vi "2b_state_sel.vi"(9 "keys pressed":T1(array[ring]), 10 "down/back":dbl, 11 "up/fwd":dbl) -> (2 "down/back":bool, 3 "up/fwd":bool)   [LabVIEW 2012]
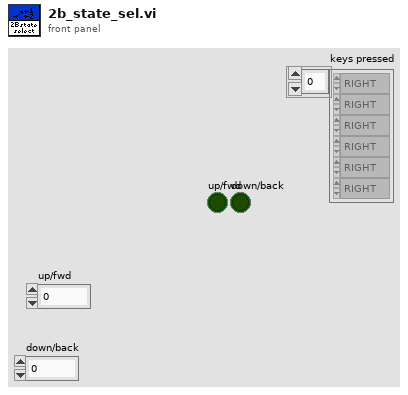
[diagram p1: front panel]
types:
  T1 = enum16{"0", "1", "2", "3", "4", "5", "6", "7", "8", "9", "A", "B", "C", "D", "E", "F", "G", "H", "I", "J", "K", "L", "M", "N", "O", "P", "Q", "R", "S", "T", "U", "V", "W", "X", "Y", "Z", "F1", "F2", "F3", "F4", "F5", "F6", "F7", "F8", "F9", "F10", "F11", "F12", "F13", "F14", "F15", "ADD", "BACK", "BACKSLASH", "CAPITAL", "COMMA", "DECIMAL", "DELETE", "DIVIDE", "DOWN", "END", "EQUALS", "ESCAPE", "GRAVE (`)", "HOME", "INSERT", "LBRACKET", "LCONTROL", "LEFT", "L ALT", "LSHIFT", "LWIN", "MINUS", "MULTIPLY", "NEXT", "NUMLOCK", "NUMPAD_0", "NUMPAD_1", "NUMPAD_2", "NUMPAD_3", "NUMPAD_4", "NUMPAD_5", "NUMPAD_6", "NUMPAD_7", "NUMPAD_8", "NUMPAD_9", "PAUSE", "PERIOD", "PRIOR (PG UP)", "RBRACKET", "RCONTROL", "RETURN", "RIGHT", "R ALT", "RSHIFT", "RWIN", "SCROLL", "SEMICOLON", "SLASH", "SPACE", "SUBTRACT", "TAB", "UP", "ENTER (num pad)", "' (quote)"}[]
  T2 = cluster{"keys pressed[0]":enum16{"0", "1", "2", "3", "4", "5", "6", "7", "8", "9", "A", "B", "C", "D", "E", "F", "G", "H", "I", "J", "K", "L", "M", "N", "O", "P", "Q", "R", "S", "T", "U", "V", "W", "X", "Y", "Z", "F1", "F2", "F3", "F4", "F5", "F6", "F7", "F8", "F9", "F10", "F11", "F12", "F13", "F14", "F15", "ADD", "BACK", "BACKSLASH", "CAPITAL", "COMMA", "DECIMAL", "DELETE", "DIVIDE", "DOWN", "END", "EQUALS", "ESCAPE", "GRAVE (`)", "HOME", "INSERT", "LBRACKET", "LCONTROL", "LEFT", "L ALT", "LSHIFT", "LWIN", "MINUS", "MULTIPLY", "NEXT", "NUMLOCK", "NUMPAD_0", "NUMPAD_1", "NUMPAD_2", "NUMPAD_3", "NUMPAD_4", "NUMPAD_5", "NUMPAD_6", "NUMPAD_7", "NUMPAD_8", "NUMPAD_9", "PAUSE", "PERIOD", "PRIOR (PG UP)", "RBRACKET", "RCONTROL", "RETURN", "RIGHT", "R ALT", "RSHIFT", "RWIN", "SCROLL", "SEMICOLON", "SLASH", "SPACE", "SUBTRACT", "TAB", "UP", "ENTER (num pad)", "' (quote)"}, "keys pressed[1]":enum16{"0", "1", "2", "3", "4", "5", "6", "7", "8", "9", "A", "B", "C", "D", "E", "F", "G", "H", "I", "J", "K", "L", "M", "N", "O", "P", "Q", "R", "S", "T", "U", "V", "W", "X", "Y", "Z", "F1", "F2", "F3", "F4", "F5", "F6", "F7", "F8", "F9", "F10", "F11", "F12", "F13", "F14", "F15", "ADD", "BACK", "BACKSLASH", "CAPITAL", "COMMA", "DECIMAL", "DELETE", "DIVIDE", "DOWN", "END", "EQUALS", "ESCAPE", "GRAVE (`)", "HOME", "INSERT", "LBRACKET", "LCONTROL", "LEFT", "L ALT", "LSHIFT", "LWIN", "MINUS", "MULTIPLY", "NEXT", "NUMLOCK", "NUMPAD_0", "NUMPAD_1", "NUMPAD_2", "NUMPAD_3", "NUMPAD_4", "NUMPAD_5", "NUMPAD_6", "NUMPAD_7", "NUMPAD_8", "NUMPAD_9", "PAUSE", "PERIOD", "PRIOR (PG UP)", "RBRACKET", "RCONTROL", "RETURN", "RIGHT", "R ALT", "RSHIFT", "RWIN", "SCROLL", "SEMICOLON", "SLASH", "SPACE", "SUBTRACT", "TAB", "UP", "ENTER (num pad)", "' (quote)"}, "keys pressed[2]":enum16{"0", "1", "2", "3", "4", "5", "6", "7", "8", "9", "A", "B", "C", "D", "E", "F", "G", "H", "I", "J", "K", "L", "M", "N", "O", "P", "Q", "R", "S", "T", "U", "V", "W", "X", "Y", "Z", "F1", "F2", "F3", "F4", "F5", "F6", "F7", "F8", "F9", "F10", "F11", "F12", "F13", "F14", "F15", "ADD", "BACK", "BACKSLASH", "CAPITAL", "COMMA", "DECIMAL", "DELETE", "DIVIDE", "DOWN", "END", "EQUALS", "ESCAPE", "GRAVE (`)", "HOME", "INSERT", "LBRACKET", "LCONTROL", "LEFT", "L ALT", "LSHIFT", "LWIN", "MINUS", "MULTIPLY", "NEXT", "NUMLOCK", "NUMPAD_0", "NUMPAD_1", "NUMPAD_2", "NUMPAD_3", "NUMPAD_4", "NUMPAD_5", "NUMPAD_6", "NUMPAD_7", "NUMPAD_8", "NUMPAD_9", "PAUSE", "PERIOD", "PRIOR (PG UP)", "RBRACKET", "RCONTROL", "RETURN", "RIGHT", "R ALT", "RSHIFT", "RWIN", "SCROLL", "SEMICOLON", "SLASH", "SPACE", "SUBTRACT", "TAB", "UP", "ENTER (num pad)", "' (quote)"}, "keys pressed[3]":enum16{"0", "1", "2", "3", "4", "5", "6", "7", "8", "9", "A", "B", "C", "D", "E", "F", "G", "H", "I", "J", "K", "L", "M", "N", "O", "P", "Q", "R", "S", "T", "U", "V", "W", "X", "Y", "Z", "F1", "F2", "F3", "F4", "F5", "F6", "F7", "F8", "F9", "F10", "F11", "F12", "F13", "F14", "F15", "ADD", "BACK", "BACKSLASH", "CAPITAL", "COMMA", "DECIMAL", "DELETE", "DIVIDE", "DOWN", "END", "EQUALS", "ESCAPE", "GRAVE (`)", "HOME", "INSERT", "LBRACKET", "LCONTROL", "LEFT", "L ALT", "LSHIFT", "LWIN", "MINUS", "MULTIPLY", "NEXT", "NUMLOCK", "NUMPAD_0", "NUMPAD_1", "NUMPAD_2", "NUMPAD_3", "NUMPAD_4", "NUMPAD_5", "NUMPAD_6", "NUMPAD_7", "NUMPAD_8", "NUMPAD_9", "PAUSE", "PERIOD", "PRIOR (PG UP)", "RBRACKET", "RCONTROL", "RETURN", "RIGHT", "R ALT", "RSHIFT", "RWIN", "SCROLL", "SEMICOLON", "SLASH", "SPACE", "SUBTRACT", "TAB", "UP", "ENTER (num pad)", "' (quote)"}, "keys pressed[4]":enum16{"0", "1", "2", "3", "4", "5", "6", "7", "8", "9", "A", "B", "C", "D", "E", "F", "G", "H", "I", "J", "K", "L", "M", "N", "O", "P", "Q", "R", "S", "T", "U", "V", "W", "X", "Y", "Z", "F1", "F2", "F3", "F4", "F5", "F6", "F7", "F8", "F9", "F10", "F11", "F12", "F13", "F14", "F15", "ADD", "BACK", "BACKSLASH", "CAPITAL", "COMMA", "DECIMAL", "DELETE", "DIVIDE", "DOWN", "END", "EQUALS", "ESCAPE", "GRAVE (`)", "HOME", "INSERT", "LBRACKET", "LCONTROL", "LEFT", "L ALT", "LSHIFT", "LWIN", "MINUS", "MULTIPLY", "NEXT", "NUMLOCK", "NUMPAD_0", "NUMPAD_1", "NUMPAD_2", "NUMPAD_3", "NUMPAD_4", "NUMPAD_5", "NUMPAD_6", "NUMPAD_7", "NUMPAD_8", "NUMPAD_9", "PAUSE", "PERIOD", "PRIOR (PG UP)", "RBRACKET", "RCONTROL", "RETURN", "RIGHT", "R ALT", "RSHIFT", "RWIN", "SCROLL", "SEMICOLON", "SLASH", "SPACE", "SUBTRACT", "TAB", "UP", "ENTER (num pad)", "' (quote)"}, "keys pressed[5]":enum16{"0", "1", "2", "3", "4", "5", "6", "7", "8", "9", "A", "B", "C", "D", "E", "F", "G", "H", "I", "J", "K", "L", "M", "N", "O", "P", "Q", "R", "S", "T", "U", "V", "W", "X", "Y", "Z", "F1", "F2", "F3", "F4", "F5", "F6", "F7", "F8", "F9", "F10", "F11", "F12", "F13", "F14", "F15", "ADD", "BACK", "BACKSLASH", "CAPITAL", "COMMA", "DECIMAL", "DELETE", "DIVIDE", "DOWN", "END", "EQUALS", "ESCAPE", "GRAVE (`)", "HOME", "INSERT", "LBRACKET", "LCONTROL", "LEFT", "L ALT", "LSHIFT", "LWIN", "MINUS", "MULTIPLY", "NEXT", "NUMLOCK", "NUMPAD_0", "NUMPAD_1", "NUMPAD_2", "NUMPAD_3", "NUMPAD_4", "NUMPAD_5", "NUMPAD_6", "NUMPAD_7", "NUMPAD_8", "NUMPAD_9", "PAUSE", "PERIOD", "PRIOR (PG UP)", "RBRACKET", "RCONTROL", "RETURN", "RIGHT", "R ALT", "RSHIFT", "RWIN", "SCROLL", "SEMICOLON", "SLASH", "SPACE", "SUBTRACT", "TAB", "UP", "ENTER (num pad)", "' (quote)"}, "keys pressed[6]":enum16{"0", "1", "2", "3", "4", "5", "6", "7", "8", "9", "A", "B", "C", "D", "E", "F", "G", "H", "I", "J", "K", "L", "M", "N", "O", "P", "Q", "R", "S", "T", "U", "V", "W", "X", "Y", "Z", "F1", "F2", "F3", "F4", "F5", "F6", "F7", "F8", "F9", "F10", "F11", "F12", "F13", "F14", "F15", "ADD", "BACK", "BACKSLASH", "CAPITAL", "COMMA", "DECIMAL", "DELETE", "DIVIDE", "DOWN", "END", "EQUALS", "ESCAPE", "GRAVE (`)", "HOME", "INSERT", "LBRACKET", "LCONTROL", "LEFT", "L ALT", "LSHIFT", "LWIN", "MINUS", "MULTIPLY", "NEXT", "NUMLOCK", "NUMPAD_0", "NUMPAD_1", "NUMPAD_2", "NUMPAD_3", "NUMPAD_4", "NUMPAD_5", "NUMPAD_6", "NUMPAD_7", "NUMPAD_8", "NUMPAD_9", "PAUSE", "PERIOD", "PRIOR (PG UP)", "RBRACKET", "RCONTROL", "RETURN", "RIGHT", "R ALT", "RSHIFT", "RWIN", "SCROLL", "SEMICOLON", "SLASH", "SPACE", "SUBTRACT", "TAB", "UP", "ENTER (num pad)", "' (quote)"}, "keys pressed[7]":enum16{"0", "1", "2", "3", "4", "5", "6", "7", "8", "9", "A", "B", "C", "D", "E", "F", "G", "H", "I", "J", "K", "L", "M", "N", "O", "P", "Q", "R", "S", "T", "U", "V", "W", "X", "Y", "Z", "F1", "F2", "F3", "F4", "F5", "F6", "F7", "F8", "F9", "F10", "F11", "F12", "F13", "F14", "F15", "ADD", "BACK", "BACKSLASH", "CAPITAL", "COMMA", "DECIMAL", "DELETE", "DIVIDE", "DOWN", "END", "EQUALS", "ESCAPE", "GRAVE (`)", "HOME", "INSERT", "LBRACKET", "LCONTROL", "LEFT", "L ALT", "LSHIFT", "LWIN", "MINUS", "MULTIPLY", "NEXT", "NUMLOCK", "NUMPAD_0", "NUMPAD_1", "NUMPAD_2", "NUMPAD_3", "NUMPAD_4", "NUMPAD_5", "NUMPAD_6", "NUMPAD_7", "NUMPAD_8", "NUMPAD_9", "PAUSE", "PERIOD", "PRIOR (PG UP)", "RBRACKET", "RCONTROL", "RETURN", "RIGHT", "R ALT", "RSHIFT", "RWIN", "SCROLL", "SEMICOLON", "SLASH", "SPACE", "SUBTRACT", "TAB", "UP", "ENTER (num pad)", "' (quote)"}, "keys pressed[8]":enum16{"0", "1", "2", "3", "4", "5", "6", "7", "8", "9", "A", "B", "C", "D", "E", "F", "G", "H", "I", "J", "K", "L", "M", "N", "O", "P", "Q", "R", "S", "T", "U", "V", "W", "X", "Y", "Z", "F1", "F2", "F3", "F4", "F5", "F6", "F7", "F8", "F9", "F10", "F11", "F12", "F13", "F14", "F15", "ADD", "BACK", "BACKSLASH", "CAPITAL", "COMMA", "DECIMAL", "DELETE", "DIVIDE", "DOWN", "END", "EQUALS", "ESCAPE", "GRAVE (`)", "HOME", "INSERT", "LBRACKET", "LCONTROL", "LEFT", "L ALT", "LSHIFT", "LWIN", "MINUS", "MULTIPLY", "NEXT", "NUMLOCK", "NUMPAD_0", "NUMPAD_1", "NUMPAD_2", "NUMPAD_3", "NUMPAD_4", "NUMPAD_5", "NUMPAD_6", "NUMPAD_7", "NUMPAD_8", "NUMPAD_9", "PAUSE", "PERIOD", "PRIOR (PG UP)", "RBRACKET", "RCONTROL", "RETURN", "RIGHT", "R ALT", "RSHIFT", "RWIN", "SCROLL", "SEMICOLON", "SLASH", "SPACE", "SUBTRACT", "TAB", "UP", "ENTER (num pad)", "' (quote)"}}
  T3 = enum16{"0", "1", "2", "3", "4", "5", "6", "7", "8", "9", "A", "B", "C", "D", "E", "F", "G", "H", "I", "J", "K", "L", "M", "N", "O", "P", "Q", "R", "S", "T", "U", "V", "W", "X", "Y", "Z", "F1", "F2", "F3", "F4", "F5", "F6", "F7", "F8", "F9", "F10", "F11", "F12", "F13", "F14", "F15", "ADD", "BACK", "BACKSLASH", "CAPITAL", "COMMA", "DECIMAL", "DELETE", "DIVIDE", "DOWN", "END", "EQUALS", "ESCAPE", "GRAVE (`)", "HOME", "INSERT", "LBRACKET", "LCONTROL", "LEFT", "L ALT", "LSHIFT", "LWIN", "MINUS", "MULTIPLY", "NEXT", "NUMLOCK", "NUMPAD_0", "NUMPAD_1", "NUMPAD_2", "NUMPAD_3", "NUMPAD_4", "NUMPAD_5", "NUMPAD_6", "NUMPAD_7", "NUMPAD_8", "NUMPAD_9", "PAUSE", "PERIOD", "PRIOR (PG UP)", "RBRACKET", "RCONTROL", "RETURN", "RIGHT", "R ALT", "RSHIFT", "RWIN", "SCROLL", "SEMICOLON", "SLASH", "SPACE", "SUBTRACT", "TAB", "UP", "ENTER (num pad)", "' (quote)"}
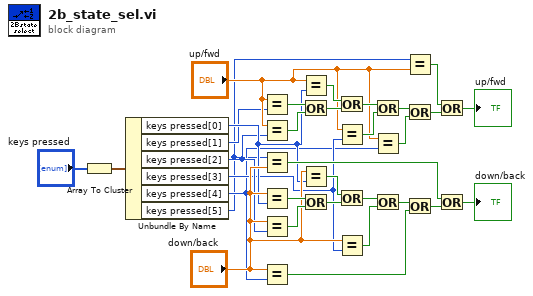
[diagram p0: block diagram]
diagram:
  n1 = Array To Cluster(array="keys pressed") -> (cluster=w7:T2)
  n2 = Unbundle By Name(w7) -> ("keys pressed[0]"=w6:T3, "keys pressed[1]"=w5:T3, "keys pressed[2]"=w4:T3, "keys pressed[3]"=w3:T3, "keys pressed[4]"=w2:T3, "keys pressed[5]"=w1:T3)
  n3 = Equal?(x="up/fwd", y=w5) -> (x = y?=w29:bool)
  n4 = Equal?(x="up/fwd", y=w4) -> (x = y?=w28:bool)
  n5 = Equal?(x=w1, y="down/back") -> (x = y?=w11:bool)
  n6 = Equal?(x="down/back", y=w6) -> (x = y?=w26:bool)
  n7 = Equal?(x="down/back", y=w4) -> (x = y?=w25:bool)
  n8 = Equal?(x="down/back", y=w2) -> (x = y?=w18:bool)
  n9 = Equal?(x="up/fwd", y=w6) -> (x = y?=w30:bool)
  n10 = Or(x=w29, y=w28) -> (x .or. y?=w32:bool)
  n11 = Equal?(x="down/back", y=w6) -> (x = y?=w27:bool)
  n12 = Or(x=w26, y=w25) -> (x .or. y?=w31:bool)
  n13 = Or(x=w30, y=w32) -> (x .or. y?=w21:bool)
  n14 = Equal?(x="up/fwd", y=w3) -> (x = y?=w22:bool)
  n15 = Or(x=w27, y=w31) -> (x .or. y?=w24:bool)
  n16 = Equal?(x="down/back", y=w3) -> (x = y?=w23:bool)
  n17 = Or(x=w21, y=w22) -> (x .or. y?=w19:bool)
  n18 = Equal?(x="up/fwd", y=w2) -> (x = y?=w20:bool)
  n19 = Or(x=w24, y=w23) -> (x .or. y?=w17:bool)
  n20 = Equal?(x=w1, y="up/fwd") -> (x = y?=w12:bool)
  n21 = Or(x=w19, y=w20) -> (x .or. y?=w16:bool)
  n22 = Or(x=w17, y=w18) -> (x .or. y?=w14:bool)
  n23 = Or(x=w12, y=w16) -> (x .or. y?=→"up/fwd":bool)
  n24 = Or(x=w11, y=w14) -> (x .or. y?=→"down/back":bool)
